vi "PicoScope6000aAdvancedTriggerSettings.vi"(0 "handle in":i16=16384, 5 "error in":errorcluster, 6 "Trigger Conditions":T7={"Channel A"=0, "Channel B"=0, "Channel C"=0, "Channel D"=0, "Channel E"=0, "Channel F"=0, "Channel G"=0, "Channel H"=0, "Port 0"=0, "Port 1"=0, "Aux"=0, "PWQ"=1, "Condition Logic"=0} {"Port 1" items=["Don't Care", "True", "False"]; "Channel H" items=["Don't Care", "True", "False"]; "Channel G" items=["Don't Care", "True", "False"]; "Channel F" items=["Don't Care", "True", "False"]; "Channel E" items=["Don't Care", "True", "False"]; "PWQ" items=["Don't Care", "True", "False"]; "Aux" items=["Don't Care", "True", "False"]; "Port 0" items=["Don't Care", "True", "False"]; "Channel D" items=["Don't Care", "True", "False"]; "Channel C" items=["Don't Care", "True", "False"]; "Channel B" items=["Don't Care", "True", "False"]; "Channel A" items=["Don't Care", "True", "False"]; "Condition Logic" items=["AND", "OR", "XOR"]}, 7 "Pulse Width Qualifier Conditions":T1={"Channel A"=1, "Channel B"=0, "Channel C"=0, "Channel D"=0, "Channel E"=0, "Channel F"=0, "Channel G"=0, "Channel H"=0, "Port 0"=0, "Port 1"=0, "Aux"=0, "Condition Logic"=0} {"Port 1" items=["Don't Care", "True", "False"]; "Channel H" items=["Don't Care", "True", "False"]; "Channel G" items=["Don't Care", "True", "False"]; "Channel F" items=["Don't Care", "True", "False"]; "Channel E" items=["Don't Care", "True", "False"]; "Aux" items=["Don't Care", "True", "False"]; "Port 0" items=["Don't Care", "True", "False"]; "Channel D" items=["Don't Care", "True", "False"]; "Channel C" items=["Don't Care", "True", "False"]; "Channel B" items=["Don't Care", "True", "False"]; "Channel A" items=["Don't Care", "True", "False"]; "Condition Logic" items=["AND", "OR", "XOR"]}, 8 "Channel Trigger Properties":T5={"Channel A Trigger Properties"={"thresholdUpper"=0, "thresholdUpperHysteresis"=0, "thresholdLower"=0, "thresholdLowerHysteresis"=0, "Threshold Mode"=0, "Direction"=2, "Available"=TRUE}, "Channel B Trigger Properties"={"thresholdUpper"=0, "thresholdUpperHysteresis"=0, "thresholdLower"=0, "thresholdLowerHysteresis"=0, "Threshold Mode"=0, "Direction"=2, "Available"=FALSE}, "Channel C Trigger Properties"={"thresholdUpper"=0, "thresholdUpperHysteresis"=0, "thresholdLower"=0, "thresholdLowerHysteresis"=0, "Threshold Mode"=0, "Direction"=2, "Available"=FALSE}, "Channel D Trigger Properties"={"thresholdUpper"=0, "thresholdUpperHysteresis"=0, "thresholdLower"=0, "thresholdLowerHysteresis"=0, "Threshold Mode"=0, "Direction"=2, "Available"=FALSE}, "Channel E Trigger Properties"={"thresholdUpper"=0, "thresholdUpperHysteresis"=0, "thresholdLower"=0, "thresholdLowerHysteresis"=0, "Threshold Mode"=0, "Direction"=2, "Available"=FALSE}, "Channel F Trigger Properties"={"thresholdUpper"=0, "thresholdUpperHysteresis"=0, "thresholdLower"=0, "thresholdLowerHysteresis"=0, "Threshold Mode"=0, "Direction"=2, "Available"=FALSE}, "Channel G Trigger Properties"={"thresholdUpper"=0, "thresholdUpperHysteresis"=0, "thresholdLower"=0, "thresholdLowerHysteresis"=0, "Threshold Mode"=0, "Direction"=2, "Available"=FALSE}, "Channel H Trigger Properties"={"thresholdUpper"=0, "thresholdUpperHysteresis"=0, "thresholdLower"=0, "thresholdLowerHysteresis"=0, "Threshold Mode"=0, "Direction"=2, "Available"=FALSE}} {"Channel H Trigger Properties"."Direction" items=["Above / Inside", "Below / Outside", "Rising / Enter", "Falling / Exit", "Rising or Falling / Enter or Exit", "Above Lower", "Below Lower", "Rising Lower", "Falling Lower", "Positive Runt", "Negative Runt"]; "Channel H Trigger Properties"."Threshold Mode" items=["Level", "Window"]; "Channel G Trigger Properties"."Direction" items=["Above / Inside", "Below / Outside", "Rising / Enter", "Falling / Exit", "Rising or Falling / Enter or Exit", "Above Lower", "Below Lower", "Rising Lower", "Falling Lower", "Positive Runt", "Negative Runt"]; "Channel G Trigger Properties"."Threshold Mode" items=["Level", "Window"]; "Channel F Trigger Properties"."Direction" items=["Above / Inside", "Below / Outside", "Rising / Enter", "Falling / Exit", "Rising or Falling / Enter or Exit", "Above Lower", "Below Lower", "Rising Lower", "Falling Lower", "Positive Runt", "Negative Runt"]; "Channel F Trigger Properties"."Threshold Mode" items=["Level", "Window"]; "Channel E Trigger Properties"."Direction" items=["Above / Inside", "Below / Outside", "Rising / Enter", "Falling / Exit", "Rising or Falling / Enter or Exit", "Above Lower", "Below Lower", "Rising Lower", "Falling Lower", "Positive Runt", "Negative Runt"]; "Channel E Trigger Properties"."Threshold Mode" items=["Level", "Window"]; "Channel D Trigger Properties"."Direction" items=["Above / Inside", "Below / Outside", "Rising / Enter", "Falling / Exit", "Rising or Falling / Enter or Exit", "Above Lower", "Below Lower", "Rising Lower", "Falling Lower", "Positive Runt", "Negative Runt"]; "Channel D Trigger Properties"."Threshold Mode" items=["Level", "Window"]; "Channel C Trigger Properties"."Direction" items=["Above / Inside", "Below / Outside", "Rising / Enter", "Falling / Exit", "Rising or Falling / Enter or Exit", "Above Lower", "Below Lower", "Rising Lower", "Falling Lower", "Positive Runt", "Negative Runt"]; "Channel C Trigger Properties"."Threshold Mode" items=["Level", "Window"]; "Channel B Trigger Properties"."Direction" items=["Above / Inside", "Below / Outside", "Rising / Enter", "Falling / Exit", "Rising or Falling / Enter or Exit", "Above Lower", "Below Lower", "Rising Lower", "Falling Lower", "Positive Runt", "Negative Runt"]; "Channel B Trigger Properties"."Threshold Mode" items=["Level", "Window"]; "Channel A Trigger Properties"."Direction" items=["Above / Inside", "Below / Outside", "Rising / Enter", "Falling / Exit", "Rising or Falling / Enter or Exit", "Above Lower", "Below Lower", "Rising Lower", "Falling Lower", "Positive Runt", "Negative Runt"]; "Channel A Trigger Properties"."Threshold Mode" items=["Level", "Window"]}, 9 "Pulse Width Qualifier Trigger Properties":T2={"Channel A Trigger Properties"={"Threshold Mode"=0, "Available"=TRUE, "Direction"=2}, "Channel B Trigger Properties"={"Threshold Mode"=0, "Available"=FALSE, "Direction"=2}, "Channel C Trigger Properties"={"Threshold Mode"=0, "Available"=FALSE, "Direction"=2}, "Channel D Trigger Properties"={"Threshold Mode"=0, "Available"=FALSE, "Direction"=2}, "Channel E Trigger Properties"={"Threshold Mode"=0, "Available"=FALSE, "Direction"=2}, "Channel F Trigger Properties"={"Threshold Mode"=0, "Available"=FALSE, "Direction"=2}, "Channel G Trigger Properties"={"Threshold Mode"=0, "Available"=FALSE, "Direction"=2}, "Channel H Trigger Properties"={"Threshold Mode"=0, "Available"=FALSE, "Direction"=2}, "Port 0 Trigger Properties"={"Threshold Mode"=0, "Available"=FALSE, "Direction"=2}, "Port 1 Trigger Properties"={"Threshold Mode"=0, "Available"=FALSE, "Direction"=2}} {"Port 1 Trigger Properties"."Direction" items=["Rising"=2, "Falling"=3, "Rising Lower"=7, "Above"=0, "Below"=1, "Rising or Falling"=4, "Falling Lower"=8, "Below Lower"=6, "Above Lower"=5]; "Port 1 Trigger Properties"."Threshold Mode" items=["Level", "Window"]; "Port 0 Trigger Properties"."Direction" items=["Rising"=2, "Falling"=3, "Rising Lower"=7, "Above"=0, "Below"=1, "Rising or Falling"=4, "Falling Lower"=8, "Below Lower"=6, "Above Lower"=5]; "Port 0 Trigger Properties"."Threshold Mode" items=["Level", "Window"]; "Channel H Trigger Properties"."Direction" items=["Rising"=2, "Falling"=3, "Rising Lower"=7, "Above"=0, "Below"=1, "Rising or Falling"=4, "Falling Lower"=8, "Below Lower"=6, "Above Lower"=5]; "Channel H Trigger Properties"."Threshold Mode" items=["Level", "Window"]; "Channel G Trigger Properties"."Direction" items=["Rising"=2, "Falling"=3, "Rising Lower"=7, "Above"=0, "Below"=1, "Rising or Falling"=4, "Falling Lower"=8, "Below Lower"=6, "Above Lower"=5]; "Channel G Trigger Properties"."Threshold Mode" items=["Level", "Window"]; "Channel F Trigger Properties"."Direction" items=["Rising"=2, "Falling"=3, "Rising Lower"=7, "Above"=0, "Below"=1, "Rising or Falling"=4, "Falling Lower"=8, "Below Lower"=6, "Above Lower"=5]; "Channel F Trigger Properties"."Threshold Mode" items=["Level", "Window"]; "Channel E Trigger Properties"."Direction" items=["Rising"=2, "Falling"=3, "Rising Lower"=7, "Above"=0, "Below"=1, "Rising or Falling"=4, "Falling Lower"=8, "Below Lower"=6, "Above Lower"=5]; "Channel E Trigger Properties"."Threshold Mode" items=["Level", "Window"]; "Channel D Trigger Properties"."Direction" items=["Rising"=2, "Falling"=3, "Rising Lower"=7, "Above"=0, "Below"=1, "Rising or Falling"=4, "Falling Lower"=8, "Below Lower"=6, "Above Lower"=5]; "Channel D Trigger Properties"."Threshold Mode" items=["Level", "Window"]; "Channel C Trigger Properties"."Direction" items=["Rising"=2, "Falling"=3, "Rising Lower"=7, "Above"=0, "Below"=1, "Rising or Falling"=4, "Falling Lower"=8, "Below Lower"=6, "Above Lower"=5]; "Channel C Trigger Properties"."Threshold Mode" items=["Level", "Window"]; "Channel B Trigger Properties"."Direction" items=["Rising"=2, "Falling"=3, "Rising Lower"=7, "Above"=0, "Below"=1, "Rising or Falling"=4, "Falling Lower"=8, "Below Lower"=6, "Above Lower"=5]; "Channel B Trigger Properties"."Threshold Mode" items=["Level", "Window"]; "Channel A Trigger Properties"."Direction" items=["Rising"=2, "Falling"=3, "Rising Lower"=7, "Above"=0, "Below"=1, "Rising or Falling"=4, "Falling Lower"=8, "Below Lower"=6, "Above Lower"=5]; "Channel A Trigger Properties"."Threshold Mode" items=["Level", "Window"]}, 10 "Digital Ports":T4 {"Digital Port  1"."Direction Channel 15" items=["Don't Care", "Low", "High", "Rising", "Falling"]; "Digital Port  1"."Direction Channel 14" items=["Don't Care", "Low", "High", "Rising", "Falling"]; "Digital Port  1"."Direction Channel 13" items=["Don't Care", "Low", "High", "Rising", "Falling"]; "Digital Port  1"."Direction Channel 12" items=["Don't Care", "Low", "High", "Rising", "Falling"]; "Digital Port  1"."Direction Channel 11" items=["Don't Care", "Low", "High", "Rising", "Falling"]; "Digital Port  1"."Direction Channel 10" items=["Don't Care", "Low", "High", "Rising", "Falling"]; "Digital Port  1"."Direction Channel 9" items=["Don't Care", "Low", "High", "Rising", "Falling"]; "Digital Port  1"."Direction Channel 8" items=["Don't Care", "Low", "High", "Rising", "Falling"]; "Digital Port  0"."Direction Channel 7" items=["Don't Care", "Low", "High", "Rising", "Falling"]; "Digital Port  0"."Direction Channel 6" items=["Don't Care", "Low", "High", "Rising", "Falling"]; "Digital Port  0"."Direction Channel 5" items=["Don't Care", "Low", "High", "Rising", "Falling"]; "Digital Port  0"."Direction Channel 4" items=["Don't Care", "Low", "High", "Rising", "Falling"]; "Digital Port  0"."Direction Channel 3" items=["Don't Care", "Low", "High", "Rising", "Falling"]; "Digital Port  0"."Direction Channel 2" items=["Don't Care", "Low", "High", "Rising", "Falling"]; "Digital Port  0"."Direction Channel 1" items=["Don't Care", "Low", "High", "Rising", "Falling"]; "Digital Port  0"."Direction Channel 0" items=["Don't Care", "Low", "High", "Rising", "Falling"]}, 11 "Pulse Width Qualifier Settings":T3 {"Pulse Width Type" items=["None", "Less Than", "Greater Than", "In Range", "Out of Range"]}, 12 "Auto Trigger (ms)":u32=1000, 13 "Trigger Delay (samples)":u64) -> (14 "handle out":i16=16384, 19 "error out":errorcluster)   [LabVIEW 2010]
doc: "This VI is an interface for the advanced trigger features of the oscilloscope.\nA simple trigger can be set using PicoScopeXXXXSettings.vi, in which case it is not necessary to use this VI."
uses:
  ps6000a.dll
panel:
  in  "Addition Trigger Properties":T6={"Ext. Trigger Properties (DO NOT USE)"={"thresholdUpper"=0, "thresholdUpperHysteresis"=0, "thresholdLower"=0, "thresholdLowerHysteresis"=0, "Threshold Mode"=0, "Direction"=2, "Available"=FALSE}, "Aux. Trigger Properties"={"thresholdUpper"=0, "thresholdUpperHysteresis"=0, "thresholdLower"=0, "thresholdLowerHysteresis"=0, "Threshold Mode"=0, "Direction"=2, "Available"=FALSE}} {"Aux. Trigger Properties"."Direction" items=["Above / Inside", "Below / Outside", "Rising / Enter", "Falling / Exit", "Rising or Falling / Enter or Exit", "Above Lower", "Below Lower", "Rising Lower", "Falling Lower", "Positive Runt", "Negative Runt"]; "Aux. Trigger Properties"."Threshold Mode" items=["Level", "Window"]; "Ext. Trigger Properties (DO NOT USE)"."Direction" items=["Above / Inside", "Below / Outside", "Rising / Enter", "Falling / Exit", "Rising or Falling / Enter or Exit", "Above Lower", "Below Lower", "Rising Lower", "Falling Lower", "Positive Runt", "Negative Runt"]; "Ext. Trigger Properties (DO NOT USE)"."Threshold Mode" items=["Level", "Window"]}
  in  "SetTrigger Info Action XOR":bool=TRUE
  out "XOR Debug Array":u32[][](array[numeric])
  in  "SetTrigger Info Action OR":bool=TRUE
  # "For Condition Logic Suggested settings;\nFor AND, XOR logic-(parallel triggers)\nUse level-type triggers (Level or Inside/outside Window Triggers)\n\nFor OR logic- (single channel)\nUse edge types (e.g. rising, falling, entering window)"
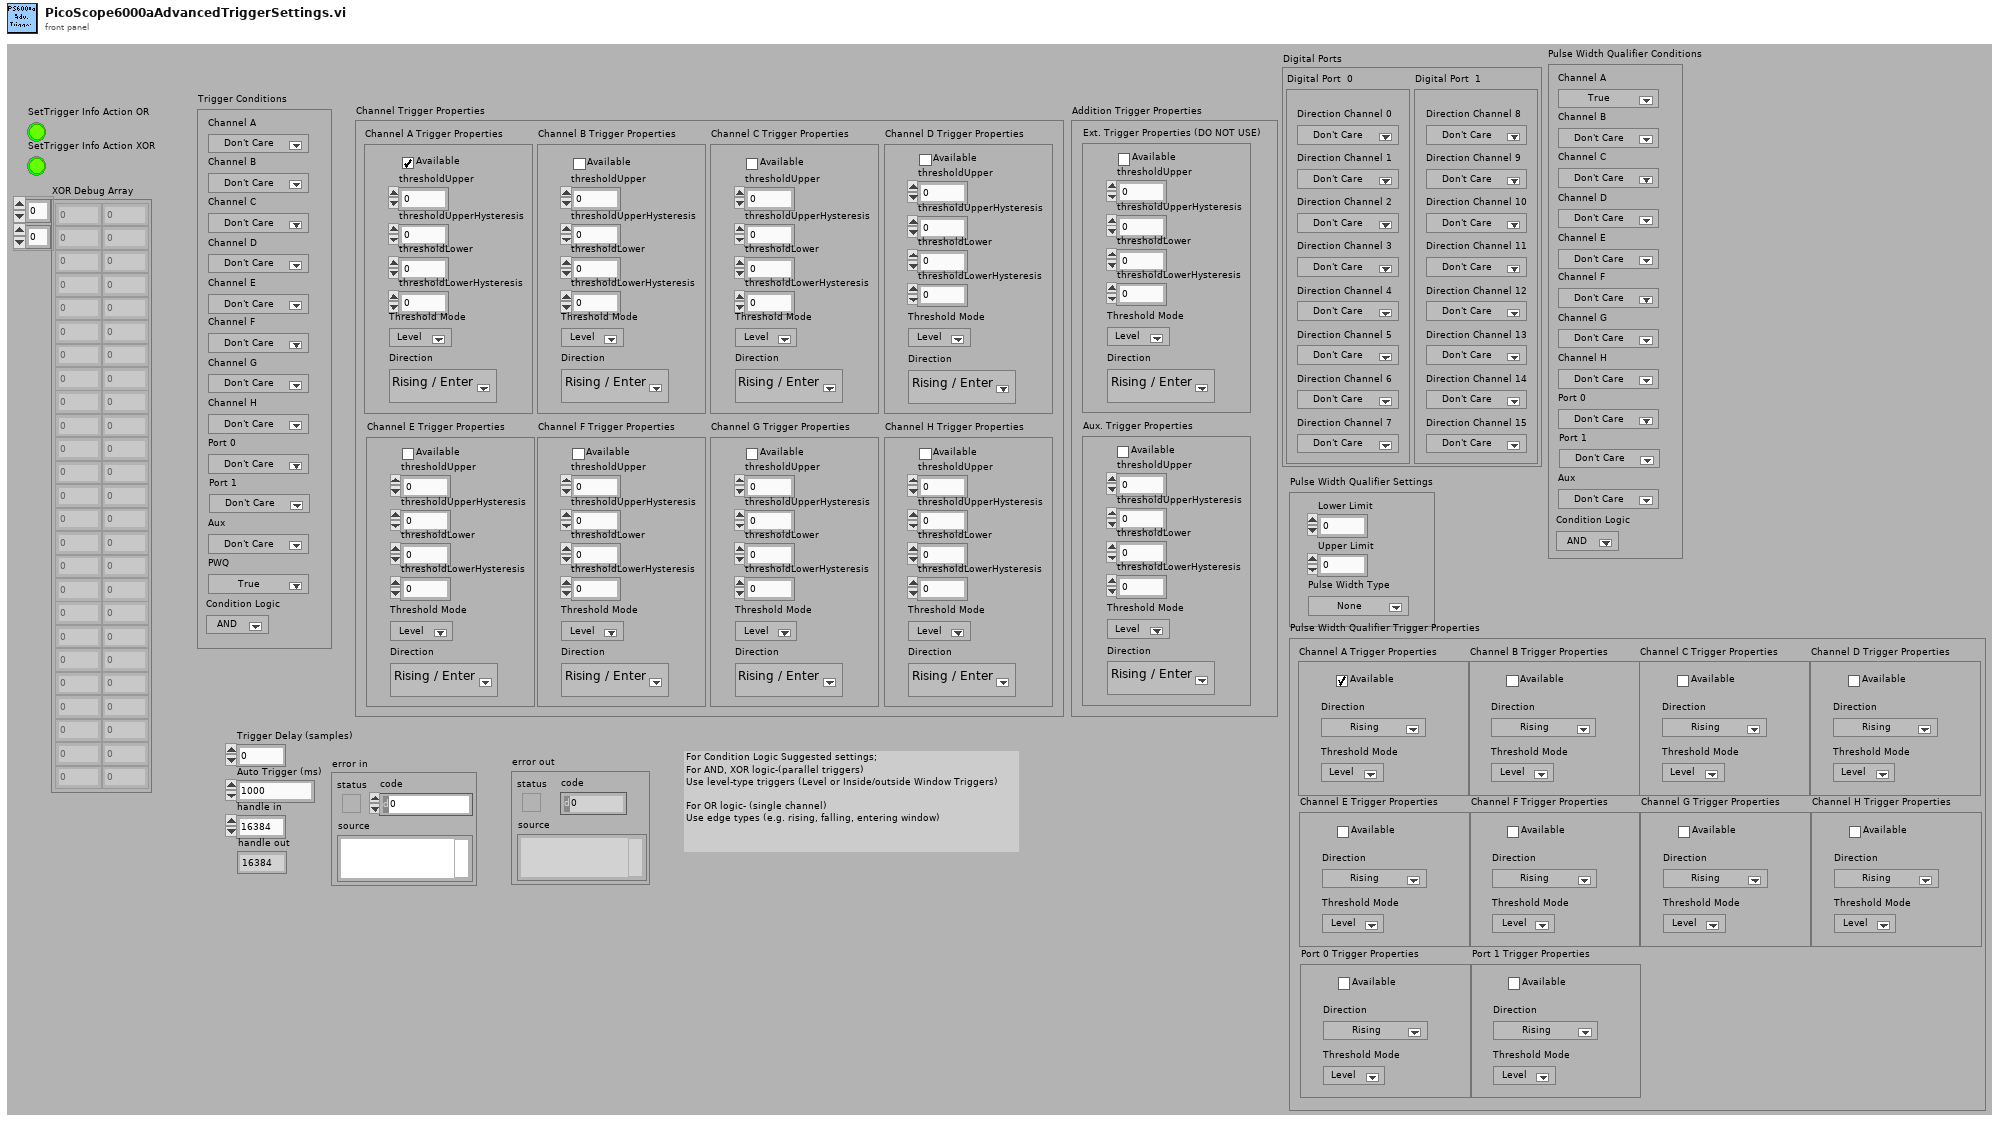
[diagram p1: front panel]
types:
  T1 = cluster{"Channel A":u16, "Channel B":u16, "Channel C":u16, "Channel D":u16, "Channel E":u16, "Channel F":u16, "Channel G":u16, "Channel H":u16, "Port 0":u16, "Port 1":u16, "Aux":u16, "Condition Logic":u16}
  T2 = cluster{"Channel A Trigger Properties":cluster{"Threshold Mode":i32, "Available":bool, "Direction":u32}, "Channel B Trigger Properties":cluster{"Threshold Mode":i32, "Available":bool, "Direction":u32}, "Channel C Trigger Properties":cluster{"Threshold Mode":i32, "Available":bool, "Direction":u32}, "Channel D Trigger Properties":cluster{"Threshold Mode":i32, "Available":bool, "Direction":u32}, "Channel E Trigger Properties":cluster{"Threshold Mode":i32, "Available":bool, "Direction":u32}, "Channel F Trigger Properties":cluster{"Threshold Mode":i32, "Available":bool, "Direction":u32}, "Channel G Trigger Properties":cluster{"Threshold Mode":i32, "Available":bool, "Direction":u32}, "Channel H Trigger Properties":cluster{"Threshold Mode":i32, "Available":bool, "Direction":u32}, "Port 0 Trigger Properties":cluster{"Threshold Mode":i32, "Available":bool, "Direction":u32}, "Port 1 Trigger Properties":cluster{"Threshold Mode":i32, "Available":bool, "Direction":u32}}
  T3 = cluster{"Lower Limit":u32, "Upper Limit":u32, "Pulse Width Type":u32}
  T4 = cluster{"Digital Port  0":cluster{"Direction Channel 0":u16, "Direction Channel 1":u16, "Direction Channel 2":u16, "Direction Channel 3":u16, "Direction Channel 4":u16, "Direction Channel 5":u16, "Direction Channel 6":u16, "Direction Channel 7":u16}, "Digital Port  1":cluster{"Direction Channel 8":u16, "Direction Channel 9":u16, "Direction Channel 10":u16, "Direction Channel 11":u16, "Direction Channel 12":u16, "Direction Channel 13":u16, "Direction Channel 14":u16, "Direction Channel 15":u16}}
  T5 = cluster{"Channel A Trigger Properties":cluster{"thresholdUpper":i16, "thresholdUpperHysteresis":u16, "thresholdLower":i16, "thresholdLowerHysteresis":u16, "Threshold Mode":i32, "Direction":i32, "Available":bool}, "Channel B Trigger Properties":cluster{"thresholdUpper":i16, "thresholdUpperHysteresis":u16, "thresholdLower":i16, "thresholdLowerHysteresis":u16, "Threshold Mode":i32, "Direction":i32, "Available":bool}, "Channel C Trigger Properties":cluster{"thresholdUpper":i16, "thresholdUpperHysteresis":u16, "thresholdLower":i16, "thresholdLowerHysteresis":u16, "Threshold Mode":i32, "Direction":i32, "Available":bool}, "Channel D Trigger Properties":cluster{"thresholdUpper":i16, "thresholdUpperHysteresis":u16, "thresholdLower":i16, "thresholdLowerHysteresis":u16, "Threshold Mode":i32, "Direction":i32, "Available":bool}, "Channel E Trigger Properties":cluster{"thresholdUpper":i16, "thresholdUpperHysteresis":u16, "thresholdLower":i16, "thresholdLowerHysteresis":u16, "Threshold Mode":i32, "Direction":i32, "Available":bool}, "Channel F Trigger Properties":cluster{"thresholdUpper":i16, "thresholdUpperHysteresis":u16, "thresholdLower":i16, "thresholdLowerHysteresis":u16, "Threshold Mode":i32, "Direction":i32, "Available":bool}, "Channel G Trigger Properties":cluster{"thresholdUpper":i16, "thresholdUpperHysteresis":u16, "thresholdLower":i16, "thresholdLowerHysteresis":u16, "Threshold Mode":i32, "Direction":i32, "Available":bool}, "Channel H Trigger Properties":cluster{"thresholdUpper":i16, "thresholdUpperHysteresis":u16, "thresholdLower":i16, "thresholdLowerHysteresis":u16, "Threshold Mode":i32, "Direction":i32, "Available":bool}}
  T6 = cluster{"Ext. Trigger Properties (DO NOT USE)":cluster{"thresholdUpper":i16, "thresholdUpperHysteresis":u16, "thresholdLower":i16, "thresholdLowerHysteresis":u16, "Threshold Mode":i32, "Direction":i32, "Available":bool}, "Aux. Trigger Properties":cluster{"thresholdUpper":i16, "thresholdUpperHysteresis":u16, "thresholdLower":i16, "thresholdLowerHysteresis":u16, "Threshold Mode":i32, "Direction":i32, "Available":bool}}
  T7 = cluster{"Channel A":u16, "Channel B":u16, "Channel C":u16, "Channel D":u16, "Channel E":u16, "Channel F":u16, "Channel G":u16, "Channel H":u16, "Port 0":u16, "Port 1":u16, "Aux":u16, "PWQ":u16, "Condition Logic":u16}
  T8 = cluster{"status":bool, "code":u32, "source":string}
  T9 = cluster{"thresholdUpper":i16, "thresholdUpperHysteresis":u16, "thresholdLower":i16, "thresholdLowerHysteresis":u16, "Threshold Mode":i32, "Direction":i32, "Available":bool}[]
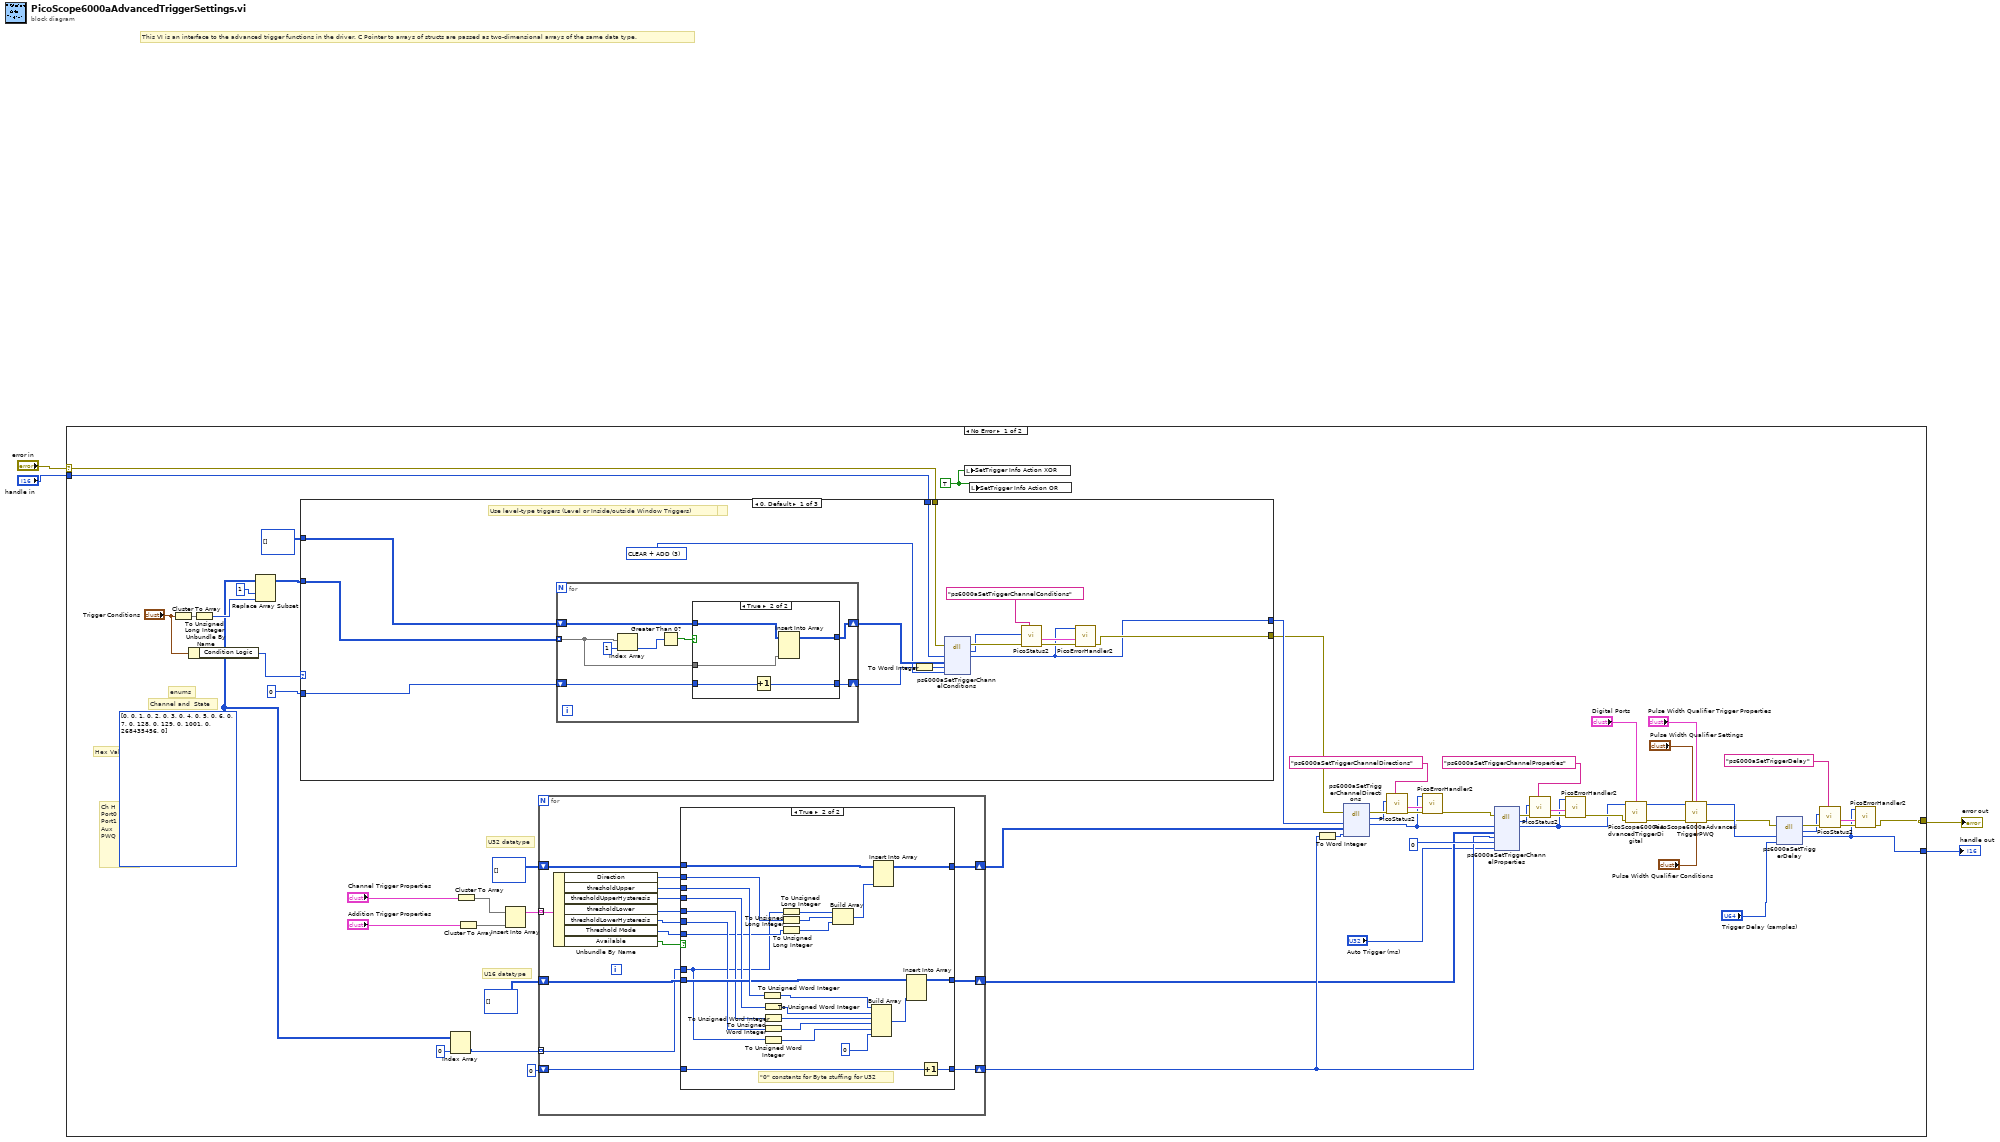
[diagram p0: block diagram]
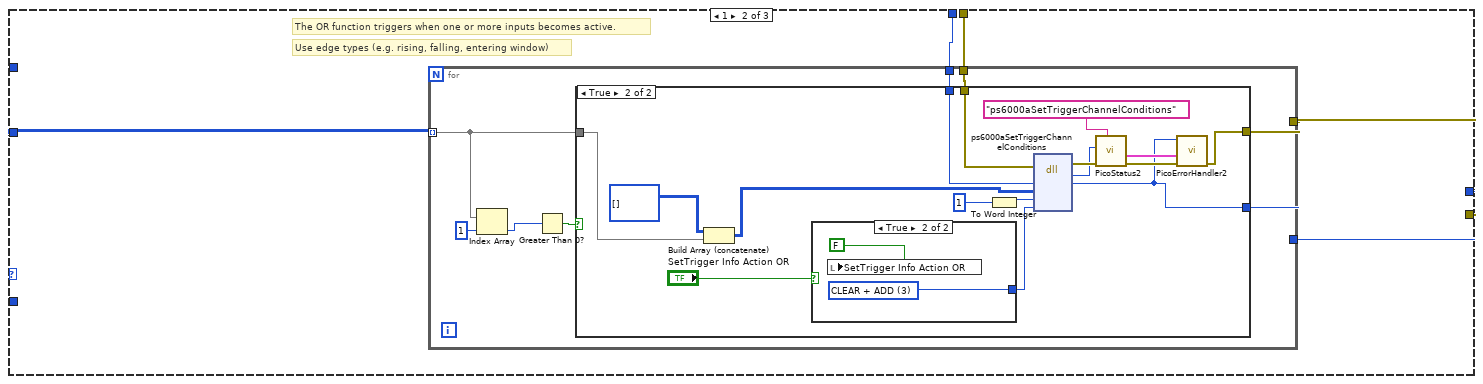
[diagram p3: hidden frame]
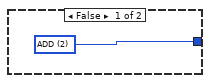
[diagram p5: hidden frame]
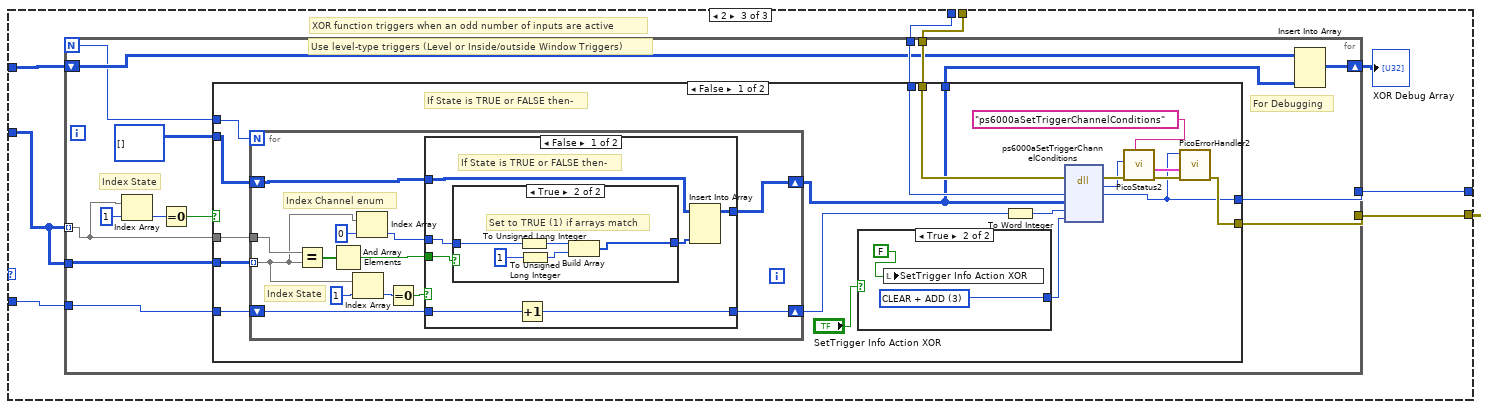
[diagram p6: hidden frame]
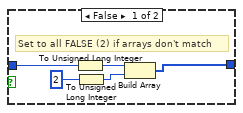
[diagram p7: hidden frame]
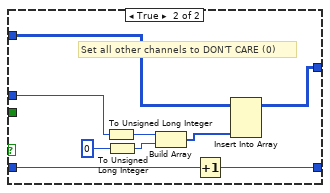
[diagram p8: hidden frame]
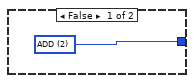
[diagram p9: hidden frame]
diagram:
  # "This VI is an interface to the advanced trigger functions in the driver. C Pointer to arrays of structs are passed as two-dimensional arrays of the same data type."
  n1 = case shown="No Error" "error in" {
    selector: "error in" -> [w46 w259]
    tunnel: "handle in" -> [w45 w260]
    tunnel: [w11 w260] -> w2
    tunnel: [w14 w259] -> w1
    frame No Error {
      w50 = TRUE ("Boolean")
      w36 = u32[][] [[0, 0], [1, 0], [2, 0], [3, 0], [4, 0], [5, 0], [6, 0], [7, 0], [128, 0], [129, 0], [1001, 0], [268435456, 0]]
      # "enums"
      # "Ch H\nPort0\nPort1\nAux\nPWQ"
      # "Channel and  State"
      # "Hex Values"
      # "U16 datatype"
      # "U32 datatype"
      n2 = Cluster To Array(cluster="Trigger Conditions") -> (array=w56:u16[])
      n3 = Unbundle By Name("Trigger Conditions") -> ("Condition Logic"=w38:u16)
      n4 = To Unsigned Long Integer(number=w56) -> (unsigned 32bit integer=w53:u32[])
      n5 = Replace Array Subset(array=w36, new element=w53, index (col)=1 ("disabled index (col)")) -> (w49:u32[][])  [unwired: 1 in]
      n6 = case shown="0, Default" w38 {
        tunnel: u32[][] [] -> [w80 _ w133]
        tunnel: i16 0 -> [w79 _ w130]
        tunnel: w46 -> [w76 w100 w137]
        tunnel: w45 -> [w75 w99 w136]
        tunnel: [w69 w98 w135] -> w26
        tunnel: [w65 w97 w134] -> w47
        tunnel: w49 -> [w72 w96 w131]
        frame 0, Default {
          w73 = u32 3 items=["CLEAR + ADD"=3, "CLEAR"=1, "ADD"=2] ("Condition Action")
          # "AND function requires both inputs to be active before it will trigger."
          # "Use level-type triggers (Level or Inside/outside Window Triggers)"
          n7 = for {
            shift-right: [w87] -> w77
            shift-left: w79 -> [w86]
            shift-right: [w85] -> w74
            shift-left: w80 -> [w88]
            tunnel: w72 -> [w83] mode=indexing
            n8 = Index Array(array=w83, index=1) -> (element=w82:u32)
            n9 = Greater Than 0?(x=w82) -> (x > 0?=w84:bool)
            n10 = case shown="True" w84 {
              tunnel: w88 -> [w90 w95]
              tunnel: [w90 w94] -> w85
              tunnel: [w89 w93] -> w87
              tunnel: w86 -> [w89 w92]
              tunnel: w83 -> [_ w91]
              frame False {
              }
              frame True {
                n11 = Increment(x=w92) -> (x+1=w93:i16)
                n12 = Insert Into Array(array=w95, new element=w91) -> (w94:u32[][])  [unwired: 2 in]
              }
            }
          }
          n13 = To Word Integer(number=w77) -> (16bit integer=w78:i16)
          n14 = dll-call lib="ps6000a.dll" fn="ps6000aSetTriggerChannelConditions" ("ps3000.dll:_ps3000_open_unit@0")(error in=w76, "handle"=w75, "conditions"=w74, "nConditions"=w78, "info"=w73) -> (error out=w67:errorcluster, "PICO_STATUS"=w66:u32, "handle"=w65:i16)  [unwired: 5 in, 1 out]
          n15 = call "PicoStatus2.vi"("PICO source"="ps6000aSetTriggerChannelConditions" ("source"), "Error in"=w67, "PICO STATUS"=w66) -> ("error out"=w71:errorcluster, "PICO_STATUS out"=w70:T8)  [unwired: 5 in]
          n16 = call "PicoErrorHandler2.vi"("error in (no error)"=w71, "PICO_STATUS in"=w70, "handle In"=w65) -> ("error out"=w69:errorcluster)  [unwired: 8 in]
        }
        frame 1 {
          # "Use edge types (e.g. rising, falling, entering window)"
          # "The OR function triggers when one or more inputs becomes active."
          n17 = for {
            tunnel: w100 -> [w108]
            tunnel: w99 -> [w107]
            tunnel: [w106] -> w98
            tunnel: [w105] -> w97
            tunnel: w96 -> [w103] mode=indexing
            n18 = Index Array(array=w103, index=1) -> (element=w102:u32)
            n19 = Greater Than 0?(x=w102) -> (x > 0?=w101:bool)
            n20 = case shown="True" w101 {
              tunnel: w108 -> [w109 w125]
              tunnel: w107 -> [w110 w124]
              tunnel: [w109 w114] -> w106
              tunnel: [w110 w115] -> w105
              tunnel: w103 -> [_ w118]
              frame False {
              }
              frame True {
                n21 = Build Array (concatenate)(u32[][] [], w118) -> (w120:u32[][])
                n22 = case shown="True" "SetTrigger Info Action OR" {
                  tunnel: [w127 w129] -> w123
                  frame False {
                    w127 = u32 2 items=["CLEAR"=1, "ADD"=2, "CLEAR + ADD"=3] ("Condition Action")
                  }
                  frame True {
                    w129 = u32 3 items=["CLEAR"=1, "ADD"=2, "CLEAR + ADD"=3] ("Condition Action")
                    n23 = local write "SetTrigger Info Action OR"(FALSE ("Boolean")) -> ()
                  }
                }
                n24 = To Word Integer(number=i16 1) -> (16bit integer=w126:i16)
                n25 = dll-call lib="ps6000a.dll" fn="ps6000aSetTriggerChannelConditions" ("ps3000.dll:_ps3000_open_unit@0")(error in=w125, "handle"=w124, "conditions"=w120, "nConditions"=w126, "info"=w123) -> (error out=w112:errorcluster, "PICO_STATUS"=w111:u32, "handle"=w115:i16)  [unwired: 5 in, 1 out]
                n26 = call "PicoStatus2.vi"("PICO source"="ps6000aSetTriggerChannelConditions" ("source"), "Error in"=w112, "PICO STATUS"=w111) -> ("error out"=w117:errorcluster, "PICO_STATUS out"=w116:T8)  [unwired: 5 in]
                n27 = call "PicoErrorHandler2.vi"("error in (no error)"=w117, "PICO_STATUS in"=w116, "handle In"=w115) -> ("error out"=w114:errorcluster)  [unwired: 8 in]
              }
            }
          }
        }
        frame 2 {
          # "Use level-type triggers (Level or Inside/outside Window Triggers)"
          # "XOR function triggers when an odd number of inputs are active"
          n28 = for {
            N -> [w145]
            tunnel: w137 -> [w152]
            tunnel: w136 -> [w151]
            tunnel: [w150] -> w135
            tunnel: [w149] -> w134
            shift-right: [w147] -> w132
            shift-left: w133 -> [w148]
            tunnel: w131 -> [w139] mode=indexing
            tunnel: w131 -> [w142]
            tunnel: w130 -> [w143]
            # "Index State"
            # "For Debugging"
            n29 = Index Array(array=w139, index=1) -> (element=w140:u32)
            n30 = Equal To 0?(x=w140) -> (x = 0?=w138:bool)
            n31 = case shown="False" w138 {
              tunnel: w152 -> [w171 w214]
              tunnel: w151 -> [w170 w215]
              tunnel: [w154 w214] -> w150
              tunnel: [w153 w215] -> w149
              tunnel: [w168 w216] -> w146
              tunnel: w145 -> [w167 _]
              tunnel: u32[][] [] -> [w166 w216]
              tunnel: w143 -> [w165 _]
              tunnel: w142 -> [w164 _]
              tunnel: w139 -> [w163 _]
              frame False {
                # "If State is TRUE or FALSE then-"
                n32 = for {
                  N: w167 -> [_]
                  shift-right: [w183] -> w169
                  shift-left: w165 -> [w184]
                  shift-right: [w172] -> w168
                  shift-left: w166 -> [w173]
                  tunnel: w163 -> [w180]
                  tunnel: w164 -> [w176] mode=indexing
                  # "Index State"
                  # "Index Channel enum"
                  n33 = Equal?(x=w180, y=w176) -> (x = y?=w174:bool[])
                  n34 = And Array Elements(Boolean array=w174) -> (logical AND=w179:bool)
                  n35 = Index Array(array=w176, index=1) -> (element=w177:u32)
                  n36 = Index Array(array=w176, index=0) -> (element=w181:u32)
                  n37 = Equal To 0?(x=w177) -> (x = 0?=w175:bool)
                  n38 = case shown="False" w175 {
                    tunnel: w184 -> [w191 w202]
                    tunnel: [w190 w203] -> w183
                    tunnel: w181 -> [w189 w206]
                    tunnel: w179 -> [w188 _]
                    tunnel: w173 -> [w187 w205]
                    tunnel: [w185 w204] -> w172
                    frame False {
                      # "If State is TRUE or FALSE then-"
                      n39 = case shown="True" w188 {
                        tunnel: [w196 w201] -> w186
                        tunnel: w189 -> [w195 w200]
                        frame False {
                          # "Set to all FALSE (2) if arrays don't match"
                          n40 = To Unsigned Long Integer(number=w195) -> (unsigned 32bit integer=w193:u32)
                          n41 = To Unsigned Long Integer(number=u32 2) -> (unsigned 32bit integer=w194:u32)
                          n42 = Build Array(w193, w194) -> (w196:u32[])
                        }
                        frame True {
                          # "Set to TRUE (1) if arrays match"
                          n43 = To Unsigned Long Integer(number=w200) -> (unsigned 32bit integer=w198:u32)
                          n44 = To Unsigned Long Integer(number=u32 1) -> (unsigned 32bit integer=w199:u32)
                          n45 = Build Array(w198, w199) -> (w201:u32[])
                        }
                      }
                      n46 = Increment(x=w191) -> (x+1=w190:i16)
                      n47 = Insert Into Array(array=w187, new element=w186) -> (w185:u32[][])  [unwired: 2 in]
                    }
                    frame True {
                      # "Set all other channels to DON'T CARE (0)"
                      n48 = To Unsigned Long Integer(number=w206) -> (unsigned 32bit integer=w208:u32)
                      n49 = To Unsigned Long Integer(number=u32 0) -> (unsigned 32bit integer=w209:u32)
                      n50 = Build Array(w208, w209) -> (w210:u32[])
                      n51 = Increment(x=w202) -> (x+1=w203:i16)
                      n52 = Insert Into Array(array=w205, new element=w210) -> (w204:u32[][])  [unwired: 2 in]
                    }
                  }
                }
                n53 = case shown="True" "SetTrigger Info Action XOR" {
                  tunnel: [w211 w213] -> w160
                  frame False {
                    w211 = u32 2 items=["CLEAR + ADD"=3, "CLEAR"=1, "ADD"=2] ("Condition Action")
                  }
                  frame True {
                    w213 = u32 3 items=["CLEAR + ADD"=3, "CLEAR"=1, "ADD"=2] ("Condition Action")
                    n54 = local write "SetTrigger Info Action XOR"(FALSE ("Boolean")) -> ()
                  }
                }
                n55 = To Word Integer(number=w169) -> (16bit integer=w162:i16)
                n56 = dll-call lib="ps6000a.dll" fn="ps6000aSetTriggerChannelConditions" ("ps3000.dll:_ps3000_open_unit@0")(error in=w171, "handle"=w170, "conditions"=w168, "nConditions"=w162, "info"=w160) -> (error out=w157:errorcluster, "PICO_STATUS"=w156:u32, "handle"=w153:i16)  [unwired: 5 in, 1 out]
                n57 = call "PicoStatus2.vi"("PICO source"="ps6000aSetTriggerChannelConditions" ("source"), "Error in"=w157, "PICO STATUS"=w156) -> ("error out"=w159:errorcluster, "PICO_STATUS out"=w158:T8)  [unwired: 5 in]
                n58 = call "PicoErrorHandler2.vi"("error in (no error)"=w159, "PICO_STATUS in"=w158, "handle In"=w153) -> ("error out"=w154:errorcluster)  [unwired: 8 in]
              }
              frame True {
              }
            }
            n59 = Insert Into Array(array=w148, new element=w146) -> (w147:u32[][])  [unwired: 2 in]
          }
          "XOR Debug Array" <- w132
        }
      }
      n60 = Index Array(array=w36, index (col)=0 ("disabled index (col)")) -> (element=w35:u32[])  [unwired: 1 in]
      n61 = Cluster To Array(cluster="Channel Trigger Properties") -> (array=w42:T9)
      n62 = Cluster To Array(cluster="Addition Trigger Properties") -> (array=w40:T9)
      n63 = Insert Into Array(array=w42, new element=w40) -> (w41:T9)  [unwired: 1 in]
      n64 = for {
        tunnel: w41 -> [w218] mode=indexing
        shift-right: [w225] -> w58
        shift-left: i16 0 -> [w224]
        shift-right: [w222] -> w54
        shift-left: u16[][] [] -> [w223]
        shift-right: [w221] -> w55
        shift-left: u32[][] [] -> [w220]
        tunnel: w35 -> [w217] mode=indexing
        n65 = Unbundle By Name(w218) -> ("Direction"=w219:i32, "thresholdUpper"=w231:i16, "thresholdUpperHysteresis"=w230:u16, "thresholdLower"=w229:i16, "thresholdLowerHysteresis"=w228:u16, "Threshold Mode"=w227:i32, "Available"=w226:bool)
        n66 = case shown="True" w226 {
          tunnel: w231 -> [_ w258]
          tunnel: w230 -> [_ w244]
          tunnel: w229 -> [_ w243]
          tunnel: w228 -> [_ w242]
          tunnel: w227 -> [_ w239]
          tunnel: w217 -> [_ w236]
          tunnel: [w234 w257] -> w225
          tunnel: w224 -> [w234 w256]
          tunnel: [w233 w254] -> w222
          tunnel: w223 -> [w233 w253]
          tunnel: [w232 w252] -> w221
          tunnel: w220 -> [w232 w251]
          tunnel: w219 -> [_ w235]
          frame False {
          }
          frame True {
            # "\"0\" constants for Byte stuffing for U32"
            n67 = To Unsigned Word Integer(number=w258) -> (unsigned 16bit integer=w246:u16)
            n68 = To Unsigned Word Integer(number=w244) -> (unsigned 16bit integer=w245:u16)
            n69 = To Unsigned Word Integer(number=w243) -> (unsigned 16bit integer=w241:u16)
            n70 = To Unsigned Word Integer(number=w242) -> (unsigned 16bit integer=w247:u16)
            n71 = To Unsigned Word Integer(number=w236) -> (unsigned 16bit integer=w238:u16)
            n72 = To Unsigned Long Integer(number=w235) -> (unsigned 32bit integer=w249:u32)
            n73 = To Unsigned Long Integer(number=w236) -> (unsigned 32bit integer=w248:u32)
            n74 = To Unsigned Long Integer(number=w239) -> (unsigned 32bit integer=w240:u32)
            n75 = Build Array(w248, w249, w240) -> (w250:u32[])
            n76 = Build Array(w246, w245, w241, w247, w238, u16 0 ("element")) -> (w255:u16[])
            n77 = Insert Into Array(array=w251, new element=w250) -> (w252:u32[][])  [unwired: 2 in]
            n78 = Insert Into Array(array=w253, new element=w255) -> (w254:u16[][])  [unwired: 2 in]
            n79 = Increment(x=w256) -> (x+1=w257:i16)
          }
        }
      }
      n80 = local write "SetTrigger Info Action XOR"(w50) -> ()
      n81 = local write "SetTrigger Info Action OR"(w50) -> ()
      n82 = To Word Integer(number=w58) -> (16bit integer=w59:i16)
      n83 = dll-call lib="ps6000a.dll" fn="ps6000aSetTriggerChannelDirections" ("ps3000.dll:_ps3000_open_unit@0")(error in=w26, "handle"=w47, "directions"=w55, "nDirections"=w59) -> (error out=w19:errorcluster, "PICO_STATUS"=w5:u32, "handle"=w8:i16)  [unwired: 4 in, 1 out]
      n84 = call "PicoStatus2.vi"("PICO source"="ps6000aSetTriggerChannelDirections" ("source"), "Error in"=w19, "PICO STATUS"=w5) -> ("error out"=w21:errorcluster, "PICO_STATUS out"=w20:T8)  [unwired: 5 in]
      n85 = call "PicoErrorHandler2.vi"("error in (no error)"=w21, "PICO_STATUS in"=w20, "handle In"=w8) -> ("error out"=w16:errorcluster)  [unwired: 8 in]
      n86 = dll-call lib="ps6000a.dll" fn="ps6000aSetTriggerChannelProperties" ("ps3000.dll:_ps3000_open_unit@0")(error in=w16, "handle"=w8, "channelProperties"=w54, "nChannelProperties"=w58, "auxOutputEnable"=i16 0, "autoTriggerMilliseconds"="Auto Trigger (ms)") -> (error out=w18:errorcluster, "PICO_STATUS"=w10:u32, "handle"=w7:i16)  [unwired: 6 in, 1 out]
      n87 = call "PicoStatus2.vi"("PICO source"="ps6000aSetTriggerChannelProperties" ("source"), "Error in"=w18, "PICO STATUS"=w10) -> ("error out"=w25:errorcluster, "PICO_STATUS out"=w24:T8)  [unwired: 5 in]
      n88 = call "PicoErrorHandler2.vi"("error in (no error)"=w25, "PICO_STATUS in"=w24, "handle In"=w7) -> ("error out"=w17:errorcluster)  [unwired: 8 in]
      n89 = call "PicoScope6000aAdvancedTriggerDigital.vi"("handle in"=w7, "Digital Ports"="Digital Ports", "error in"=w17) -> ("handle out"=w34:i16, "error out"=w33:errorcluster)  [unwired: 11 in]
      n90 = call "PicoScope6000aAdvancedTriggerPWQ.vi"("handle in"=w34, "Pulse Width Qualifier Settings"="Pulse Width Qualifier Settings", "Pulse Width Qualifier Trigger Properties"="Pulse Width Qualifier Trigger Properties", "error in"=w33, "Pulse Width Qualifier Conditions"="Pulse Width Qualifier Conditions") -> ("handle out"=w32:i16, "error out"=w31:errorcluster)  [unwired: 9 in]
      n91 = dll-call lib="ps6000a.dll" fn="ps6000aSetTriggerDelay" ("ps3000.dll:_ps3000_open_unit@0")(error in=w31, "handle"=w32, "delay"="Trigger Delay (samples)") -> (error out=w15:errorcluster, "PICO_STATUS"=w12:u32, "handle"=w11:i16)  [unwired: 3 in, 1 out]
      n92 = call "PicoStatus2.vi"("PICO source"="ps6000aSetTriggerDelay" ("source"), "Error in"=w15, "PICO STATUS"=w12) -> ("error out"=w23:errorcluster, "PICO_STATUS out"=w22:T8)  [unwired: 5 in]
      n93 = call "PicoErrorHandler2.vi"("error in (no error)"=w23, "PICO_STATUS in"=w22, "handle In"=w11) -> ("error out"=w14:errorcluster)  [unwired: 8 in]
    }
    frame Error {
    }
  }
  "handle out" <- w2
  "error out" <- w1
